vi "0~1随机数发生器2D（dbl).vi"(8 "Error In":errorcluster caption="错误输入", 9 "Clol":i32, 10 "Row":i32) -> (0 "Error Out":errorcluster caption="错误输出", 3 "Rand(0~1) 2D":dbl[][](array[numeric]))   [LabVIEW 2013]
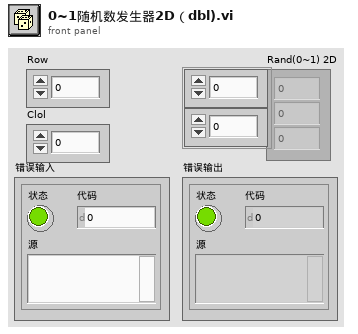
[diagram p1: front panel]
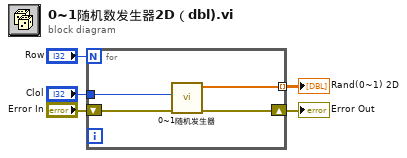
[diagram p0: block diagram]
diagram:
  n1 = for {
    N: "Row" -> [_]
    shift-right: [w8] -> w4
    shift-left: "Error In" -> [w9]
    tunnel: [w7] -> w3 mode=indexing
    tunnel: "Clol" -> [w6]
    n2 = call-poly "0~1随机发生器.vi"("Error In"=w9, "Length"=w6) -> ("Error Out"=w8:errorcluster, "Rand(0~1) 1D"=w7:dbl[])  [unwired: 8 in]
  }
  "Error Out" <- w4
  "Rand(0~1) 2D" <- w3
